vi "dfd_DFXP_Carry (vector).vi"(9 "High 64":i64[](array[numeric]), 10 "Low 64":u64[](array[numeric]), 11 "Num":i16) -> (3 "carries":u64[](array[numeric]))   [LabVIEW 2017, in "NI_DigFilter_FXP.lvlib"]
uses:
  <vilib>/addons/Digital Filter Design/NI_DigFilter_FXP.lvlib
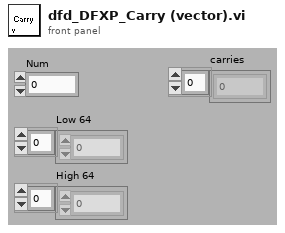
[diagram p1: front panel]
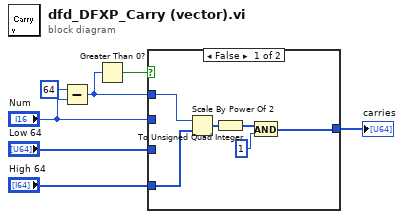
[diagram p0: block diagram]
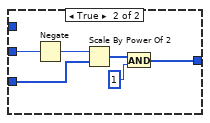
[diagram p2: hidden frame]
diagram:
  n1 = Subtract(x=i16 64 ("y"), y="Num") -> (x-y=w4:i16)
  n2 = Greater Than 0?(x=w4) -> (x > 0?=w5:bool)
  n3 = case shown="False" w5 {
    tunnel: "Low 64" -> [_ w19]
    tunnel: "High 64" -> [w12 _]
    tunnel: "Num" -> [_ w18]
    tunnel: [w9 w14] -> w1
    tunnel: w4 -> [w8 _]
    frame False {
      n4 = Scale By Power Of 2(n=w8, x=w12) -> (x*2^n=w13:i64[])
      n5 = To Unsigned Quad Integer(1:w13) -> (0:w10:u64[])
      n6 = And(x=w10, y=u64 1) -> (x .and. y?=w9:u64[])
    }
    frame True {
      n7 = Negate(x=w18) -> (-x=w17:i16)
      n8 = Scale By Power Of 2(n=w17, x=w19) -> (x*2^n=w15:u64[])
      n9 = And(x=w15, y=u64 1) -> (x .and. y?=w14:u64[])
    }
  }
  "carries" <- w1
